vi "lfieldpanel_DO_dynamic_subtraction.vi"(5 "savepath":path, 6 "num_frames":i32, 7 "Log data":bool, 8 "error in (no error)":errorcluster, 9 "notes":string, 10 "Integrate_sensor":bool, 11 "lightfield_panel in":refnum<class "lightfield_panel.lvclass">) -> (0 "error out":errorcluster, 3 "lightfield_panel out":refnum<class "lightfield_panel.lvclass">)   [LabVIEW 2015, in "lightfield_panel.lvclass"]
uses:
  lightfield_panel.lvclass
  lightfield/lightfield_class.lvclass
  Stage Class/thorlabs_filter_wheel/thorlabs_FW102C.lvclass
  UI/panel_class/panel.lvclass
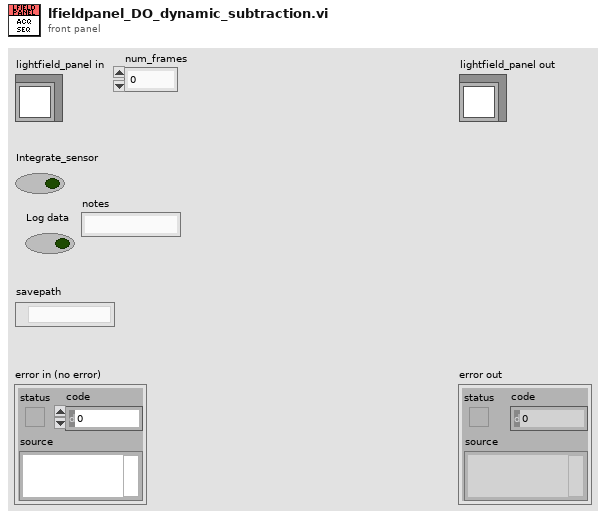
[diagram p1: front panel]
types:
  T1 = cluster{"Image":dbl[][][], "Frame Size":cluster{"F":i32, "Y":i32, "X":i32}}
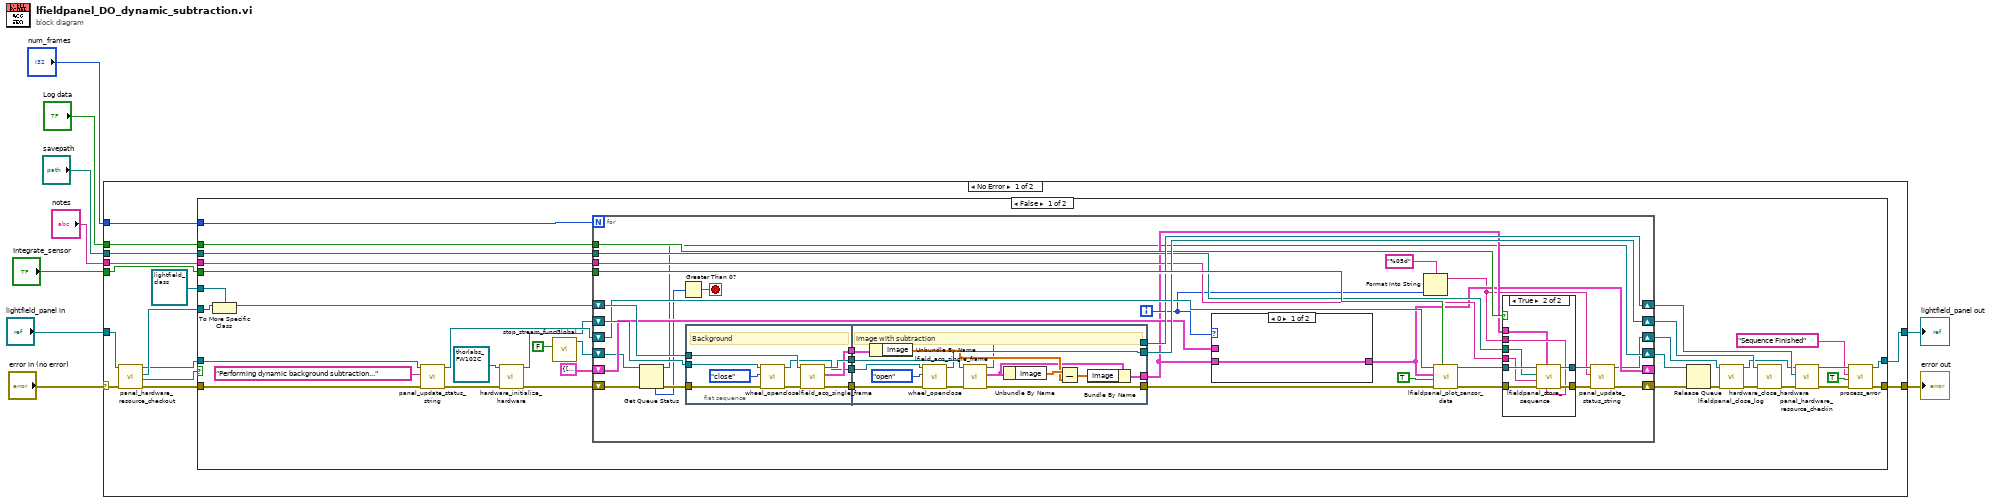
[diagram p0: block diagram]
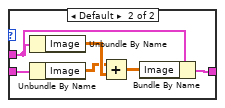
[diagram p2: hidden frame]
diagram:
  n1 = case shown="No Error" "error in (no error)" {
    selector: "error in (no error)" -> [w23 w134]
    tunnel: [w17 w134] -> w6
    tunnel: [w16 w133] -> w8
    tunnel: "lightfield_panel in" -> [w15 w133]
    tunnel: "Integrate_sensor" -> [w14 _]
    tunnel: "Log data" -> [w13 _]
    tunnel: "savepath" -> [w12 _]
    tunnel: "notes" -> [w11 _]
    tunnel: "num_frames" -> [w10 _]
    frame No Error {
      n2 = call "panel_hardware_resource_checkout.vi"("error in (no error)"=w23, "panel in"=w15) -> ("error out"=w19:errorcluster, "timed out?"=w22:bool, "hardware.lvclass"=w20:refnum<class "hardware.lvclass">, "panel out"=w18:refnum<class "lightfield_panel.lvclass">)  [unwired: 6 in]
      n3 = case shown="False" w22 {
        tunnel: refnum<class "lightfield_class.lvclass"> refnum ("lightfield_class.lvclass") -> [w57 _]
        tunnel: w20 -> [w56 _]
        tunnel: w19 -> [w46 w131]
        tunnel: w18 -> [w44 w132]
        tunnel: [w53 w131] -> w17
        tunnel: [w52 w132] -> w16
        tunnel: w14 -> [w47 _]
        tunnel: w13 -> [w36 _]
        tunnel: w12 -> [w35 _]
        tunnel: w11 -> [w34 _]
        tunnel: w10 -> [w40 _]
        frame False {
          n4 = To More Specific Class(target class=w57, reference=w56) -> (specific class reference=w49:refnum<class "lightfield_class.lvclass">)  [unwired: 1 in, 1 out]
          n5 = call-dynamic "panel_update_status_string.vi"("error in (no error)"=w46, "String"="Performing dynamic background subtraction...", "lightfield_panel in"=w44) -> ("error out"=w42:errorcluster, "lightfield_panel out"=w45:refnum<class "lightfield_panel.lvclass">)  [unwired: 7 in]
          n6 = call-dynamic "hardware_initialize_hardware.vi"("error in (no error)"=w42, "thorlabs_FW102C in"=refnum<class "thorlabs_FW102C.lvclass"> refnum) -> ("error out"=w39:errorcluster, "thorlabs_FW102C out"=w38:refnum<class "thorlabs_FW102C.lvclass">)  [unwired: 8 in]
          n7 = call "stop_stream_funcGlobal.vi"("write?"=FALSE) -> ("queue out 2"=w27:refnum<queue>)  [unwired: 10 in]
          n8 = for {
            N: w40 -> [_]
            tunnel: w47 -> [w90]
            shift-right: [w79] -> w48
            shift-left: w49 -> [w87]
            shift-right: [w59] -> w31
            shift-left: w45 -> [w80]
            shift-right: [w61] -> w26
            shift-left: w39 -> [w67]
            shift-right: [w82] -> w37
            shift-left: w38 -> [w88]
            tunnel: w36 -> [w76]
            tunnel: w35 -> [w75]
            tunnel: w34 -> [w74]
            shift-right: [w69] -> _
            shift-left: T1 {"Image"=[], "Frame Size"={"F"=0, "Y"=0, "X"=0}} ("image_data") -> [w71]
            shift-right: [w63] -> w25
            shift-left: w27 -> [w68]
            i -> [w72]
            stop <- w64 stop-if-true
            n9 = Get Queue Status(queue=w68, error in (no error)=w67) -> (queue out=w63:refnum<queue>, error out=w66:errorcluster, # elements in queue=w65:i32)  [unwired: 1 in, 5 out]
            n10 = Greater Than 0?(x=w65) -> (x > 0?=w64:bool)
            n11 = flat-sequence {
              tunnel: w66 -> [w113]
              tunnel: w88 -> [w111]
              tunnel: w87 -> [w109]
              tunnel: [w116] -> w86
              tunnel: [w115] -> w85
              tunnel: [w114] -> w84
              tunnel: [w108] -> w83
              tunnel: [w118] -> w70
              tunnel: w86 -> [w126]
              tunnel: w85 -> [w128]
              tunnel: w84 -> [w123]
              tunnel: w83 -> [w127]
              tunnel: [w125] -> w82
              tunnel: [w124] -> w81
              tunnel: [w117] -> w79
              frame #0 {
                # "Background"
                n12 = call "wheel_openclose.vi"("error in (no error)"=w113, "action"=enum16{"open", "close"}."close", "thorlabs_FW102C in"=w111) -> ("error out"=w112:errorcluster, "thorlabs_FW102C out"=w108:refnum<class "thorlabs_FW102C.lvclass">)  [unwired: 7 in]
                n13 = call "lfield_acq_single_frame.vi"("error in (no error)"=w112, "lightfield_class in"=w109) -> ("error out"=w115:errorcluster, "image_data"=w114:T1, "lightfield_class out"=w116:refnum<class "lightfield_class.lvclass">)  [unwired: 7 in]
              }
              frame #1 {
                # "Image with subtraction"
                n14 = Unbundle By Name(w123) -> ("Image"=w121:dbl[][][])
                n15 = call "wheel_openclose.vi"("error in (no error)"=w128, "action"=enum16{"open", "close"}."open", "thorlabs_FW102C in"=w127) -> ("error out"=w130:errorcluster, "thorlabs_FW102C out"=w125:refnum<class "thorlabs_FW102C.lvclass">)  [unwired: 7 in]
                n16 = call "lfield_acq_single_frame.vi"("error in (no error)"=w130, "lightfield_class in"=w126) -> ("error out"=w124:errorcluster, "image_data"=w120:T1, "lightfield_class out"=w117:refnum<class "lightfield_class.lvclass">)  [unwired: 7 in]
                n17 = Unbundle By Name(w120) -> ("Image"=w122:dbl[][][])
                n18 = Subtract(x=w122, y=w121) -> (x-y=w119:dbl[][][])
                n19 = Bundle By Name(cluster=w120, "Image"=w119) -> (w118:T1)
              }
            }
            n20 = case shown="0" w72 {
              tunnel: w71 -> [_ w94]
              tunnel: w70 -> [w91 w97]
              tunnel: [w91 w92] -> w69
              frame 0 {
              }
              frame Default {
                n21 = Unbundle By Name(w94) -> ("Image"=w96:dbl[][][])
                n22 = Unbundle By Name(w97) -> ("Image"=w95:dbl[][][])
                n23 = Add(x=w95, y=w96) -> (x+y=w93:dbl[][][])
                n24 = Bundle By Name(cluster=w94, "Image"=w93) -> (w92:T1)
              }
            }
            n25 = Format Into String(format string="%05d", w72) -> (resulting string=w58:string)  [unwired: 2 in, 1 out]
            n26 = call "lfieldpanel_plot_sensor_data.vi"("Integrate"=w90, "error in (no error)"=w81, "First_time?"=TRUE, "image_data"=w69, "lightfield_panel in"=w80) -> ("error out"=w78:errorcluster, "lightfield_panel out"=w77:refnum<class "lightfield_panel.lvclass">)  [unwired: 5 in]
            n27 = case shown="True" w76 {
              tunnel: w78 -> [w98 w107]
              tunnel: [w98 w106] -> w62
              tunnel: w77 -> [w99 w105]
              tunnel: [w99 w104] -> w60
              tunnel: w75 -> [_ w103]
              tunnel: w74 -> [_ w102]
              tunnel: w58 -> [_ w101]
              tunnel: w70 -> [_ w100]
              frame False {
              }
              frame True {
                n28 = call "lfieldpanel_store_sequence.vi"("dset_name"=w101, "image_data"=w100, "error in (no error)"=w107, "notes"=w102, "Path"=w103, "lightfield_panel in"=w105) -> ("error out"=w106:errorcluster, "lightfield_panel out"=w104:refnum<class "lightfield_panel.lvclass">)  [unwired: 4 in]
              }
            }
            n29 = call-dynamic "panel_update_status_string.vi"("error in (no error)"=w62, "String"=w58, "lightfield_panel in"=w60) -> ("error out"=w61:errorcluster, "lightfield_panel out"=w59:refnum<class "lightfield_panel.lvclass">)  [unwired: 7 in]
          }
          n30 = Release Queue(queue=w25, error in (no error)=w26) -> (error out=w24:errorcluster)  [unwired: 1 in, 2 out]
          n31 = call "lfieldpanel_close_log.vi"("error in (no error)"=w24, "lightfield_panel in"=w31) -> ("error out"=w33:errorcluster, "lightfield_panel out"=w30:refnum<class "lightfield_panel.lvclass">)  [unwired: 8 in]
          n32 = call-dynamic "hardware_close_hardware.vi"("error in (no error)"=w33, "thorlabs_FW102C in"=w37) -> ("error out"=w32:errorcluster)  [unwired: 8 in, 1 out]
          n33 = call "panel_hardware_resource_checkin.vi"("error in (no error)"=w32, "hardware.lvclass"=w48, "panel in"=w30) -> ("error out"=w54:errorcluster, "panel out"=w55:refnum<class "lightfield_panel.lvclass">)  [unwired: 7 in]
          n34 = call "process_error.vi"("error in (no error)"=w54, "Update Status"=TRUE, "No Error Message"="Sequence Finished", "lightfield_panel in"=w55) -> ("error out"=w53:errorcluster, "lightfield_panel out"=w52:refnum<class "lightfield_panel.lvclass">)  [unwired: 6 in]
        }
        frame True {
        }
      }
    }
    frame Error {
    }
  }
  "error out" <- w6
  "lightfield_panel out" <- w8
